vi "绝对路径.vi"(1 "相对路径":string) -> (0 "绝对路径":path)   [LabVIEW 2020]
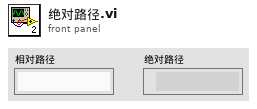
[diagram p1: front panel]
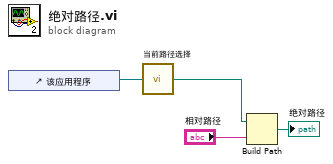
[diagram p0: block diagram]
diagram:
  n1 = control-ref of="该应用程序"() -> (w1:refnum<vi>)
  n2 = call "当前路径选择.vi"("本应用程序"=w1) -> ("当前路径"=w3:path)
  n3 = Build Path(base path=w3, name or relative path="相对路径") -> (appended path=→"绝对路径":path)
